vi "Get All Path Sets.vi"(10 "Start":cluster{"Row":i32, "Column":i32}, 11 "Grid":string[][](array[string])) -> (3 "Guard Positions":set{cluster{i32, "index of element":i32}}(c389))   [LabVIEW 2024]
uses:
  ENUM_Direction.ctl
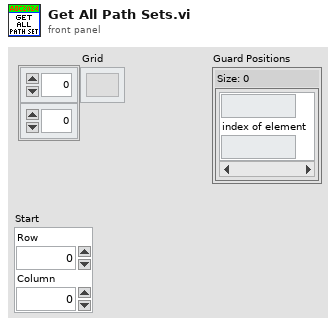
[diagram p1: front panel]
types:
  T1 = typedef "ENUM_Direction.ctl" = enum16{"Up;-1,0", "Right;0,1", "Down;1,0", "Left;0,-1"}
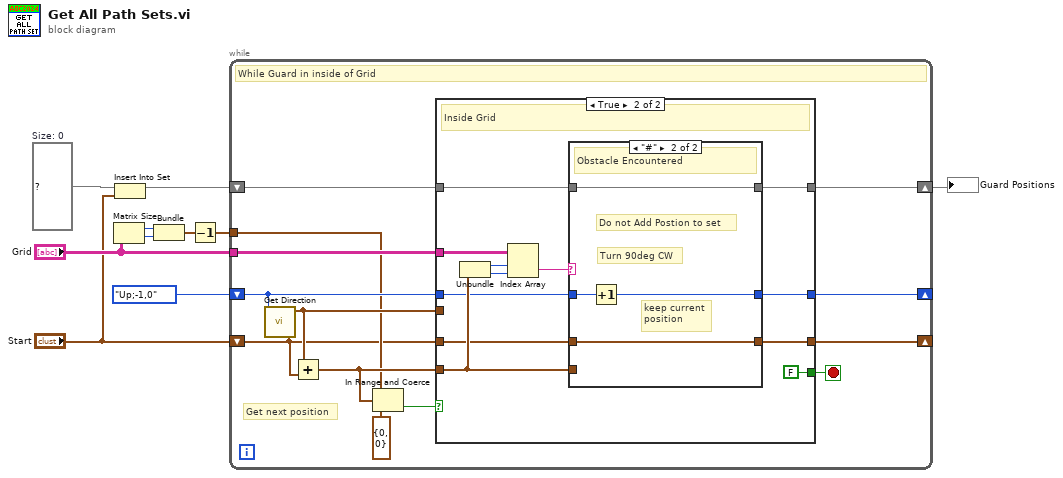
[diagram p0: block diagram]
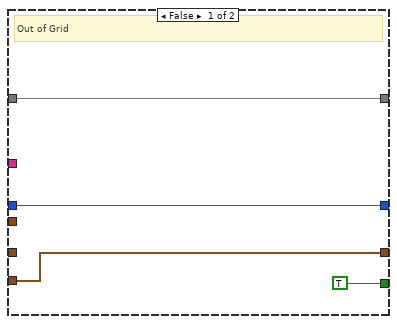
[diagram p2: hidden frame]
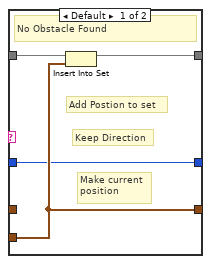
[diagram p3: hidden frame]
diagram:
  w1 = set{cluster{i32, "index of element":i32}} {}  # Size: 0
  n1 = Matrix Size(0:"Grid") -> (1:w4:i32, 2:w5:i32)
  n2 = Insert Into Set(10:"Start", 11:w1) -> (3:w2:set{cluster{i32, "index of element":i32}})  [unwired: 1 out]
  n3 = Bundle("number of columns"=w4, "matrix"=w5) -> (w7:cluster{"number of columns":i32, "matrix":i32})  [unwired: 1 in]
  n4 = Decrement(x=w7) -> (x-1=w9:cluster{"number of columns":i32, "matrix":i32})
  n5 = while {
    tunnel: "Grid" -> [w23]
    shift-right: [w19] -> _
    shift-left: "Start" -> [w11]
    shift-right: [w17] -> _
    shift-left: ENUM_Direction."Up;-1,0" ("Direction") -> [w18]
    shift-right: [w21] -> w10
    shift-left: w2 -> [w22]
    tunnel: w9 -> [w15]
    stop <- w12 stop-if-true
    # "Get next position"
    # "While Guard in inside of Grid"
    n6 = call "Get Direction.vi"("Direction"=w18) -> ("Direction"=w20:cluster{"Numeric":i32, "Numeric":i32})  [unwired: 10 in]
    n7 = Add(x=w20, y=w11) -> (x+y=w16:cluster{i32, i32})
    n8 = In Range and Coerce(upper limit=w15, x=w16, lower limit=cluster{"number of columns":i32, "matrix":i32} {"number of columns"=0, "matrix"=0}) -> (In Range?=w13:bool)  [unwired: 1 out]
    n9 = case shown="True" w13 {
      tunnel: w23 -> [_ w39]
      tunnel: w22 -> [w27 w35]
      tunnel: [w27 w34] -> w21
      tunnel: w16 -> [w25 w33]
      tunnel: w20 -> [_ _]
      tunnel: [w25 w32] -> w19
      tunnel: w18 -> [w26 w31]
      tunnel: [w26 w30] -> w17
      tunnel: [TRUE FALSE] -> w12
      tunnel: w11 -> [_ w28]
      frame False {
        # "Out of Grid"
      }
      frame True {
        # "Inside Grid"
        n10 = Unbundle(w33) -> (w38:i32, w37:i32)
        n11 = Index Array(array=w39, index (row)=w38, index (col)=w37) -> (element=w36:string)
        n12 = case shown="\"#\"" w36 {
          tunnel: w35 -> [w43 w47]
          tunnel: [w42 w47] -> w34
          tunnel: w33 -> [w41 _]
          tunnel: [w41 w44] -> w32
          tunnel: w31 -> [w40 w46]
          tunnel: [w40 w45] -> w30
          tunnel: w28 -> [_ w44]
          frame Default {
            # "Make current\nposition"
            # "Keep Direction"
            # "Add Postion to set"
            # "No Obstacle Found"
            n13 = Insert Into Set(10:w41, 11:w43) -> (3:w42:set{cluster{i32, "index of element":i32}})  [unwired: 1 out]
          }
          frame "#" {
            # "keep current\nposition"
            # "Do not Add Postion to set"
            # "Turn 90deg CW"
            # "Obstacle Encountered"
            n14 = Increment(x=w46) -> (x+1=w45:T1)
          }
        }
      }
    }
  }
  "Guard Positions" <- w10
